vi "Parse Any Cluster.vi"(8 "error in (no error)":errorcluster, 10 "JSON In":string, 11 "Cluster in":variant) -> (0 "error out":errorcluster, 3 "Cluster out":variant)   [LabVIEW 2018]
uses:
  <vilib>/JDP Science/JSONtext/Next JSON Value.vi
  <vilib>/JDP Science/JSONtext/String Subset.vi
  <vilib>/JDP Science/JSONtext/Parsing/Advance past next JSON Value (inlined COPY).vi
  <vilib>/JDP Science/JSONtext/Parsing/Advance past whitespace.vi
  <vilib>/JDP Science/JSONtext/Parsing/Advance past String.vi
  <vilib>/JDP Science/JSONtext/Parsing/Advance past Number.vi
  <vilib>/JDP Science/JSONtext/Parsing/Advance past Line Ending.vi
  <vilib>/JDP Science/JSONtext/Parsing/Parse Full Path or Item Name.vi
  <vilib>/JDP Science/JSONtext/Parsing/Advance past Array.vi
  <vilib>/JDP Science/JSONtext/Parsing/Advance past Object.vi
  <vilib>/JDP Science/JSONtext/support/Error Cluster From Code.vi
  <vilib>/JDP Science/JSONtext/Offset/Find Item Locations by Path.vi
  <vilib>/Utility/Data Type/NI_Data Type.lvlib
  <vilib>/JDP Science/JSONtext/JSONtext.lvlib
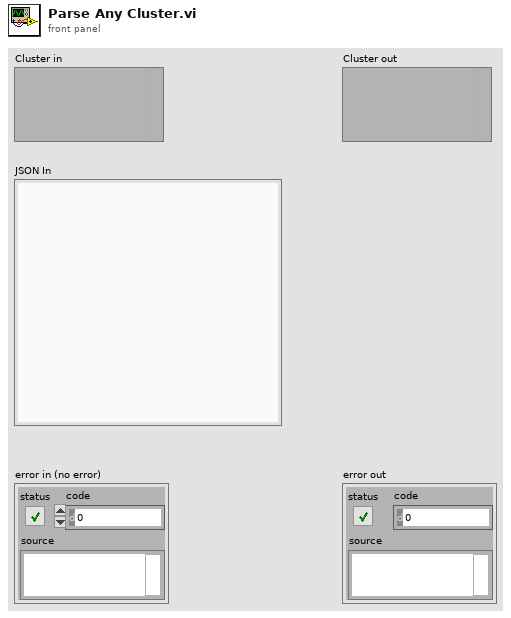
[diagram p1: front panel]
types:
  T1 = typedef "NI_Data Type.lvlib/Data Type.ctl" = enum8{"Invalid Type", "Void", "I8", "I16", "I32", "I64", "U8", "U16", "U32", "U64", "Single Float", "Double Float", "Extended Float", "Single Complex", "Double Complex", "Extended Complex", "Enum U8", "Enum U16", "Enum U32", "Enum U64", "Single Float With Unit", "Double Float With Unit", "Extended Float With Unit", "Single Complex with Unit", "Double Complex with Unit", "Extended Complex with Unit", "Boolean", "String", "Path", "Picture", "Tag", "Array", "Cluster", "Variant", "LV Variant", "Waveform", "Timestamp", "Digital Waveform", "Digital Data", "ExpressData", "Refnum", "External Data", "VI", "Poly VI", "LabVIEW Class Instance", "Fixed Point"}
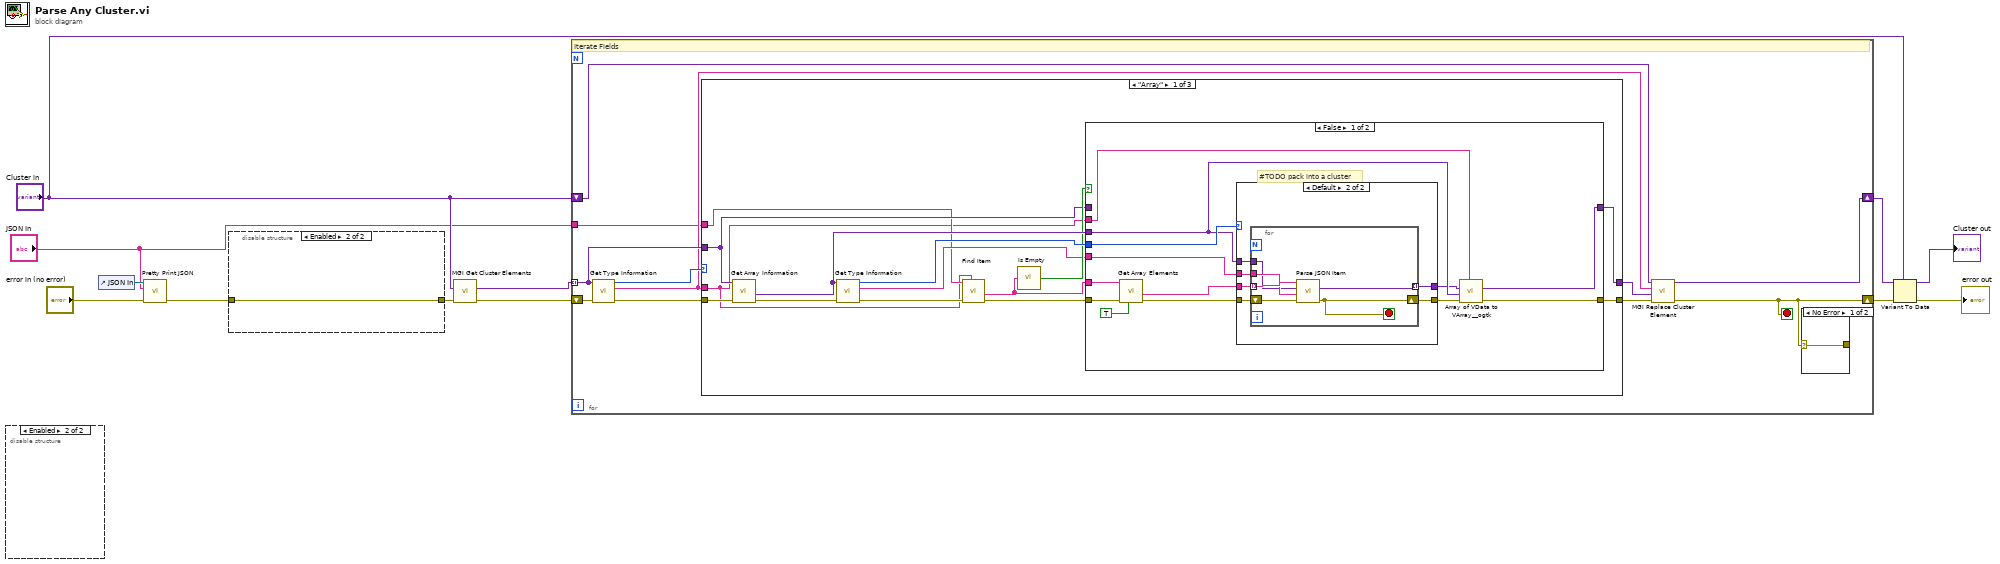
[diagram p0: block diagram]
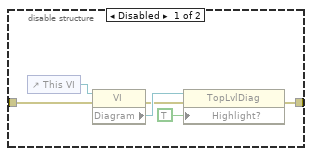
[diagram p2: hidden frame]
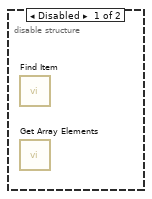
[diagram p3: hidden frame]
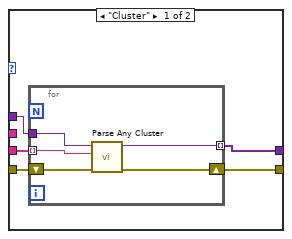
[diagram p5: hidden frame]
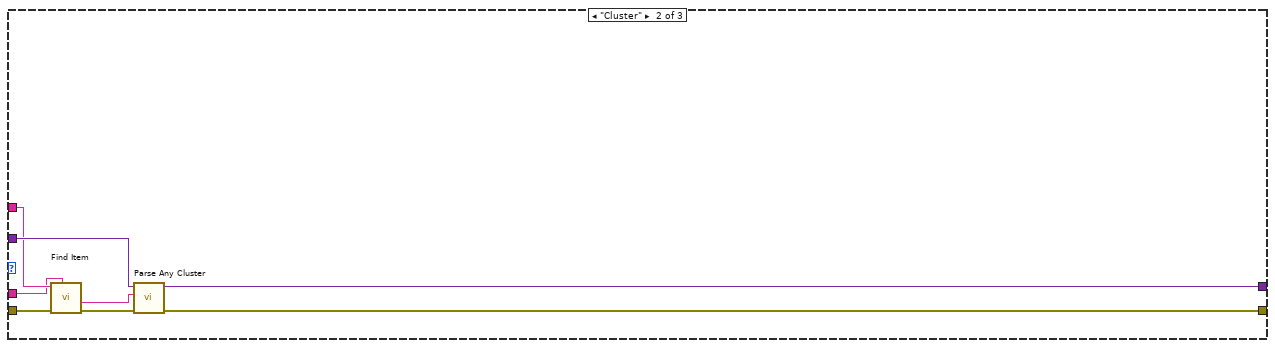
[diagram p7: hidden frame]
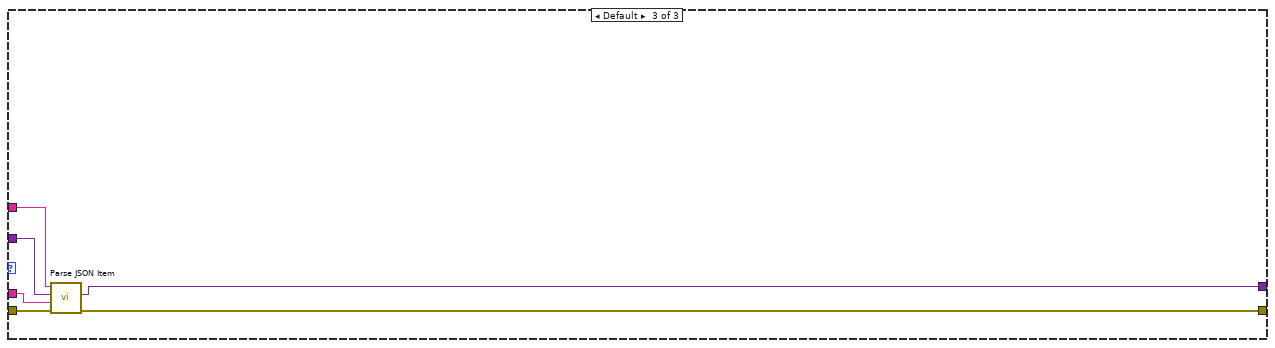
[diagram p8: hidden frame]
diagram:
  n1 = disable-structure shown="Enabled" {
    frame Disabled {
      n2 = call <vilib>:"Find Item.vi"() -> ()  [unwired: 8 in, 4 out]
      n3 = call <vilib>:"Get Array Elements.vi"() -> ()  [unwired: 9 in, 3 out]
    }
    frame Enabled {
    }
  }
  n4 = control-ref of="JSON In"() -> (w4:refnum<vi>)
  n5 = call "Pretty Print JSON.vi"("error in (no error)"="error in (no error)", "JSON in"="JSON In", "String in"=w4) -> ("error out"=w1:errorcluster)  [unwired: 8 in]
  n6 = disable-structure shown="Enabled" {
    disable-tunnel: w1 -> [w15 w19]
    disable-tunnel: [w14 w19] -> w5
    frame Disabled {
      n7 = control-ref of="This VI"() -> (w18:refnum<vi>)
      n8 = property class="VI"(reference=w18, error in=w15) -> (error out=w13:errorcluster, "Diagram"=w17:refnum<vi>)  [unwired: 1 out]
      n9 = property class="TopLvlDiag"(reference=w17, error in=w13, "Highlight?"=TRUE ("Highlight Execution?")) -> (error out=w14:errorcluster)  [unwired: 1 out]
    }
    frame Enabled {
    }
  }
  n10 = call <userlib>:"MGI Get Cluster Elements.vi"("Error In"=w5, "Cluster"="Cluster in") -> ("Error Out"=w7:errorcluster, "Cluster Elements"=w6:variant[])  [unwired: 8 in]
  n11 = for {
    tunnel: "JSON In" -> [w20]
    tunnel: w6 -> [w22] mode=indexing
    shift-right: [w23] -> w10
    shift-left: w7 -> [w30]
    shift-right: [w27] -> w8
    shift-left: "Cluster in" -> [w28]
    stop <- w23 stop-if-true
    # "Iterate Fields"
    n12 = call <vilib>:"Get Type Information.vi"("error in (no error)"=w30, "Variant"=w22) -> ("error out"=w29:errorcluster, "Name"=w21:string, "Type"=w24:T1)  [unwired: 5 in, 2 out]
    n13 = case shown="\"Array\"" w24 {
      tunnel: w20 -> [w34 w90 w97]
      tunnel: w29 -> [w46 w87 w96]
      tunnel: w22 -> [w36 w91 w94]
      tunnel: w21 -> [w33 w89 w93]
      tunnel: [w42 w84 w92] -> w26
      tunnel: [w41 w85 w95] -> w25
      frame "Array" {
        n14 = call <vilib>:"Get Array Information.vi"("error in (no error)"=w46, "Variant"=w36) -> ("error out"=w43:errorcluster, "Array Element Data Type"=w44:variant)  [unwired: 6 in, 2 out]
        n15 = call <vilib>:"Get Type Information.vi"("error in (no error)"=w43, "Variant"=w44) -> ("error out"=w40:errorcluster, "Name"=w35:string, "Type"=w45:T1)  [unwired: 5 in, 2 out]
        n16 = call <vilib>:"Find Item.vi"("$Path or Item Name"=w33, "error in (no error)"=w40, "JSON"=w34) -> ("error out"=w39:errorcluster, "<JSON>"=w38:string)  [unwired: 5 in, 2 out]
        n17 = call <vilib>:"Is Empty.vi"("JSON"=w38) -> ("Empty"=w37:bool)  [unwired: 4 in]
        n18 = case shown="False" w37 {
          tunnel: w45 -> [w59 _]
          tunnel: w44 -> [w52 _]
          tunnel: [w50 w82] -> w42
          tunnel: [w48 w83] -> w41
          tunnel: w39 -> [w57 w83]
          tunnel: w38 -> [w58 _]
          tunnel: w36 -> [_ w82]
          tunnel: w35 -> [w54 _]
          tunnel: w33 -> [w47 _]
          frame False {
            # "#TODO pack into a cluster"
            n19 = call <vilib>:"Get Array Elements.vi"("Pass non-arrays"=TRUE, "error in (no error)"=w57, "JSON"=w58) -> ("error out"=w56:errorcluster, "<JSON>"=w55:string[])  [unwired: 6 in, 1 out]
            n20 = case shown="Default" w59 {
              tunnel: w52 -> [w64 w73]
              tunnel: w56 -> [w62 w71]
              tunnel: [w60 w72] -> w51
              tunnel: w55 -> [w63 w75]
              tunnel: [w61 w70] -> w49
              tunnel: w54 -> [_ w74]
              frame "Cluster" {
                n21 = for {
                  tunnel: w64 -> [w69]
                  tunnel: w63 -> [w68] mode=indexing
                  shift-right: [w66] -> w61
                  shift-left: w62 -> [w67]
                  tunnel: [w65] -> w60 mode=indexing
                  n22 = call "Parse Any Cluster.vi"("error in (no error)"=w67, "JSON In"=w68, "Cluster in"=w69) -> ("error out"=w66:errorcluster, "Cluster out"=w65:variant)  [unwired: 7 in]
                }
              }
              frame Default {
                n23 = for {
                  tunnel: w75 -> [w81] mode=indexing
                  tunnel: w74 -> [w80]
                  tunnel: w73 -> [w76]
                  tunnel: [w77] -> w72 mode=indexing
                  shift-right: [w78] -> w70
                  shift-left: w71 -> [w79]
                  stop <- w78 stop-if-true
                  n24 = call "Parse JSON Item.vi"("error in (no error)"=w79, "Name"=w80, "Variant in"=w76, "JSON In"=w81) -> ("error out"=w78:errorcluster, "Variant out"=w77:variant)  [unwired: 6 in]
                }
              }
            }
            n25 = call <userlib>:"Array of VData to VArray__ogtk.vi"("Array Name"=w47, "error in (no error)"=w49, "Element Type (when empty)"=w52, "1D Array of VData"=w51) -> ("error out"=w48:errorcluster, "VArray"=w50:variant)  [unwired: 6 in]
          }
          frame True {
            # "Empty Array"
          }
        }
      }
      frame "Cluster" {
        n26 = call <vilib>:"Find Item.vi"("$Path or Item Name"=w89, "error in (no error)"=w87, "JSON"=w90) -> ("error out"=w86:errorcluster, "<JSON>"=w88:string)  [unwired: 5 in, 2 out]
        n27 = call "Parse Any Cluster.vi"("error in (no error)"=w86, "JSON In"=w88, "Cluster in"=w91) -> ("error out"=w85:errorcluster, "Cluster out"=w84:variant)  [unwired: 7 in]
      }
      frame Default {
        n28 = call "Parse JSON Item.vi"("error in (no error)"=w96, "Name"=w93, "Variant in"=w94, "JSON In"=w97) -> ("error out"=w95:errorcluster, "Variant out"=w92:variant)  [unwired: 6 in]
      }
    }
    n29 = call <userlib>:"MGI Replace Cluster Element.vi"("Error In"=w25, "Data"=w26, "Name"=w21, "Cluster In"=w28) -> ("Error Out"=w23:errorcluster, "Cluster Out"=w27:variant)  [unwired: 5 in, 1 out]
    n30 = case shown="No Error" w23 {
      selector: w23 -> [w31 w32]
      tunnel: [w31 w32] -> _
      frame No Error {
      }
      frame Error {
      }
    }
  }
  n31 = Variant To Data(error in=w10, type="Cluster in", Variant=w8) -> (data=→"Cluster out":variant, error out=→"error out":errorcluster)
